vi "Drive_Speed_Read(EEPRM).vi"(5 "baud rate (9600)":u32=115200 caption="보 전송속도(9600)", 6 "Axis":u16(ring) items=["X", "Y"], 7 "Drive Speed Number":u16(ring) items=["Drive Speed 1", "Drive Speed 2", "Drive Speed 3", "Drive Speed 4"], 8 "Port":refnum<visa-resource-name>="COM4" caption="VISA 리소스 이름") -> (1 "Spped":u32, 2 "에러 출력":errorcluster, 3 "VISA 리소스 이름 출력":refnum<visa-resource-name>, 4 "Read Buffer":string)   [LabVIEW 2016]
uses:
  <vilib>/Instr/_visa.llb/VISA Configure Serial Port (Instr).vi
  <vilib>/Instr/_visa.llb/VISA Flush IO Buffer Mask.ctl
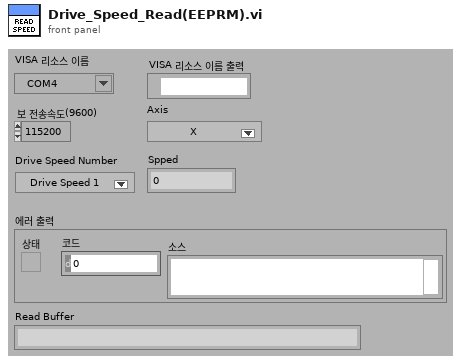
[diagram p1: front panel]
types:
  T1 = typedef "VISA Flush IO Buffer Mask.ctl" = u16
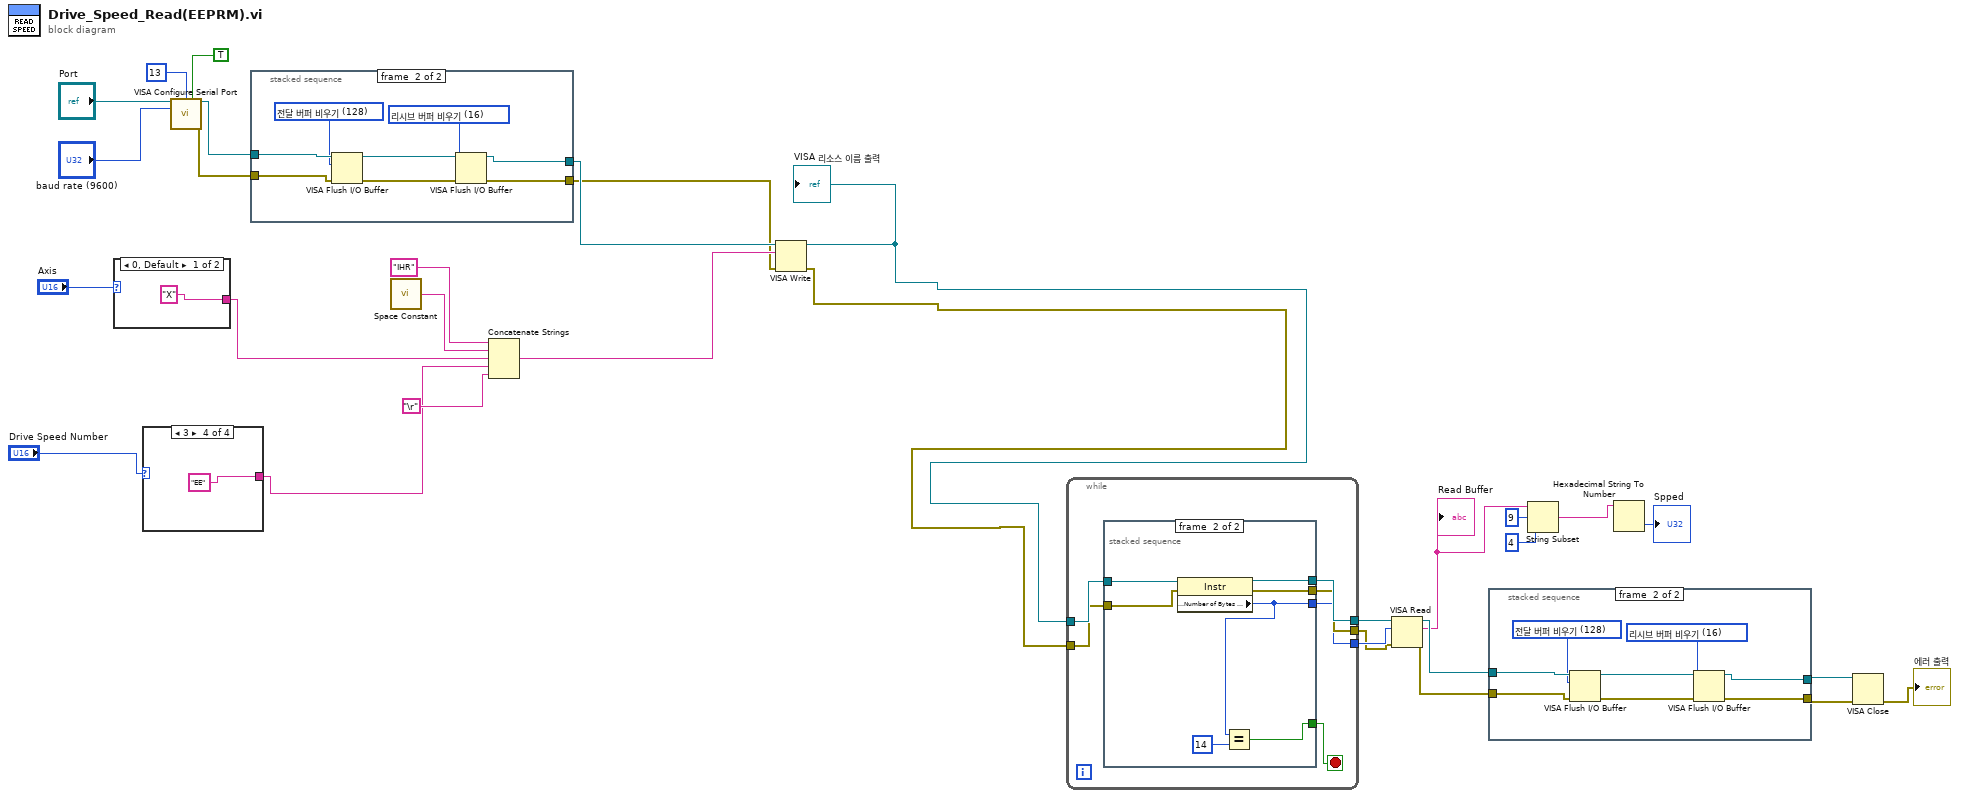
[diagram p0: block diagram]
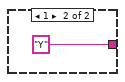
[diagram p2: hidden frame]
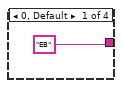
[diagram p3: hidden frame]
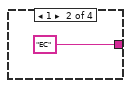
[diagram p4: hidden frame]
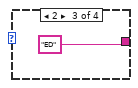
[diagram p5: hidden frame]
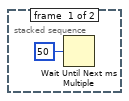
[diagram p6: hidden frame]
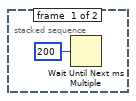
[diagram p7: hidden frame]
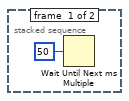
[diagram p8: hidden frame]
diagram:
  n1 = case shown="0, Default" "Axis" {
    tunnel: ["X" ("문자열") "Y" ("문자열")] -> w1
    frame 0, Default {
    }
    frame 1 {
    }
  }
  n2 = case shown="3" "Drive Speed Number" {
    tunnel: ["EB" ("문자열") "EC" ("문자열") "ED" ("문자열") "EE" ("문자열")] -> w8
    frame 0, Default {
    }
    frame 1 {
    }
    frame 2 {
    }
    frame 3 {
    }
  }
  n3 = call-poly "VISA Configure Serial Port"("VISA resource name"="Port", "termination char\n(0xA = '\\n' = LF)"=i16 13 ("termination char\n(0xA = '\\n' = LF)"), "Enable Termination\nChar (T)"=TRUE ("Enable Termination\nChar (T)"), "baud rate (9600)"="baud rate (9600)") -> ("VISA resource name out"=w24:refnum<visa-resource-name>, "error out"=w23:errorcluster)  [unwired: 10 in]
  n4 = stacked-sequence {
    tunnel: w24 -> [_ w46]
    tunnel: w23 -> [_ w45]
    tunnel: [_ w41] -> w22
    tunnel: [_ w40] -> w21
    frame #0 {
      n5 = Wait Until Next ms Multiple(millisecond multiple=u32 50 ("ms 배수")) -> ()  [unwired: 1 out]
    }
    frame #1 {
      w39 = T1 16 items=["리시브 버퍼 비우기"=16, "전달 버퍼 디바이스에 쓰기"=32, "리시브 버퍼 비우기(I/O 없음)"=64, "전달 버퍼 비우기"=128] ("Mask")
      w44 = T1 128 items=["리시브 버퍼 비우기"=16, "전달 버퍼 디바이스에 쓰기"=32, "리시브 버퍼 비우기(I/O 없음)"=64, "전달 버퍼 비우기"=128] ("Mask")
      n6 = VISA Flush I/O Buffer(VISA resource name=w46, mask (16)=w44, error in (no error)=w45) -> (VISA resource name out=w43:refnum<visa-resource-name>, error out=w42:errorcluster)
      n7 = VISA Flush I/O Buffer(VISA resource name=w43, mask (16)=w39, error in (no error)=w42) -> (VISA resource name out=w41:refnum<visa-resource-name>, error out=w40:errorcluster)
    }
  }
  n8 = call <vilib>:"Space Constant.vi"() -> ("String"=w29:string)
  n9 = Concatenate Strings("IHR" ("버퍼 쓰기"), w29, w1, w8, "\r") -> (w30:string)
  n10 = VISA Write(VISA resource name=w22, write buffer=w30, error in (no error)=w21) -> (VISA resource name out=w12:refnum<visa-resource-name>, error out=w11:errorcluster)  [unwired: 1 out]
  "VISA 리소스 이름 출력" <- w12
  n11 = while {
    tunnel: w12 -> [w52]
    tunnel: w11 -> [w51]
    tunnel: [w50] -> w19
    tunnel: [w47] -> w14
    tunnel: [w49] -> w13
    stop <- w48 stop-if-true
    n12 = stacked-sequence {
      tunnel: w52 -> [_ w60]
      tunnel: w51 -> [_ w59]
      tunnel: [_ w58] -> w50
      tunnel: [_ w57] -> w49
      tunnel: [_ w55] -> w48
      tunnel: [_ w54] -> w47
      frame #0 {
        n13 = Wait Until Next ms Multiple(millisecond multiple=u32 200 ("ms 배수")) -> ()  [unwired: 1 out]
      }
      frame #1 {
        n14 = property class="Instr"(reference=w60, error in=w59) -> (reference out=w58:refnum<visa-resource-name>, error out=w57:errorcluster, "Serial Settings:Number of Bytes at Serial Port"=w54:u32)
        n15 = Equal?(x=w54, y=u32 14) -> (x = y?=w55:bool)
      }
    }
  }
  n16 = VISA Read(VISA resource name=w19, byte count=w14, error in (no error)=w13) -> (VISA resource name out=w18:refnum<visa-resource-name>, read buffer=w7:string, error out=w17:errorcluster)  [unwired: 1 out]
  "Read Buffer" <- w7
  n17 = stacked-sequence {
    tunnel: w18 -> [_ w69]
    tunnel: w17 -> [_ w68]
    tunnel: [_ w64] -> w16
    tunnel: [_ w63] -> w15
    frame #0 {
      n18 = Wait Until Next ms Multiple(millisecond multiple=u32 50 ("ms 배수")) -> ()  [unwired: 1 out]
    }
    frame #1 {
      w62 = T1 16 items=["리시브 버퍼 비우기"=16, "전달 버퍼 디바이스에 쓰기"=32, "리시브 버퍼 비우기(I/O 없음)"=64, "전달 버퍼 비우기"=128] ("Mask")
      w67 = T1 128 items=["리시브 버퍼 비우기"=16, "전달 버퍼 디바이스에 쓰기"=32, "리시브 버퍼 비우기(I/O 없음)"=64, "전달 버퍼 비우기"=128] ("Mask")
      n19 = VISA Flush I/O Buffer(VISA resource name=w69, mask (16)=w67, error in (no error)=w68) -> (VISA resource name out=w66:refnum<visa-resource-name>, error out=w65:errorcluster)
      n20 = VISA Flush I/O Buffer(VISA resource name=w66, mask (16)=w62, error in (no error)=w65) -> (VISA resource name out=w64:refnum<visa-resource-name>, error out=w63:errorcluster)
    }
  }
  n21 = String Subset(string=w7, offset (0)=9 ("오프셋(0)"), length (rest)=4 ("길이(나머지)")) -> (substring=w4:string)
  n22 = Hexadecimal String To Number(string=w4) -> (number=→"Spped":u32)  [unwired: 2 in, 1 out]
  n23 = VISA Close(VISA resource name=w16, error in (no error)=w15) -> (error out=→"에러 출력":errorcluster)
